vi "Exercises_6-1.vi"() -> ()   [LabVIEW 2014]
uses:
  <vilib>/Utility/file.llb/Write To Spreadsheet File (DBL).vi
  <vilib>/Analysis/NI_AALBase.lvlib
panel:
  out "Waveform Graph":dbl[][](graph)
  out "Table":string[][](table)
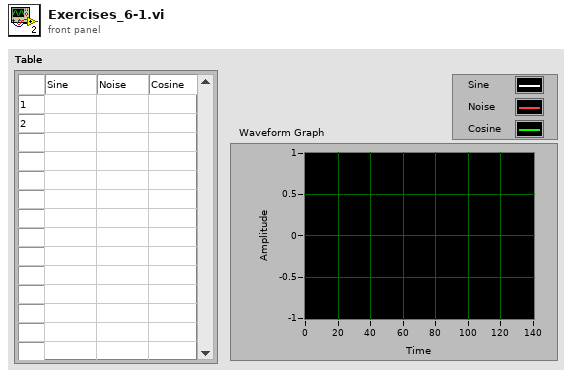
[diagram p1: front panel]
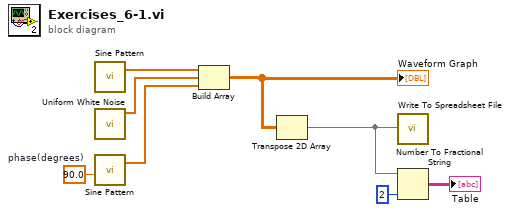
[diagram p0: block diagram]
diagram:
  w2 = 90.0  # phase(degrees)
  n1 = call <vilib>:"Sine Pattern.vi"() -> ("Sinusoidal Pattern"=w3:dbl[])  [unwired: 4 in, 1 out]
  n2 = call <vilib>:"Uniform White Noise.vi"() -> ("uniform white noise"=w8:dbl[])  [unwired: 10 in, 1 out]
  n3 = call <vilib>:"Sine Pattern.vi"("phase(degrees)"=w2) -> ("Sinusoidal Pattern"=w4:dbl[])  [unwired: 3 in, 1 out]
  n4 = Build Array "Build Array"(w3, w8, w4) -> (w5:dbl[][])
  "Waveform Graph" <- w5
  n5 = Transpose 2D Array(2D array=w5) -> (transposed array=w1:dbl[][])
  n6 = call-poly <vilib>:"Write To Spreadsheet File.vi"("2D data"=w1) -> ()  [unwired: 7 in, 1 out]
  n7 = Number To Fractional String(number=w1, precision (6)=i16 2) -> (F-format string=→"Table":string[][])  [unwired: 2 in]
